vi "Find Execution Tests From AllTests.vi"(8 "error in":errorcluster, 10 "Test Tags to Execute":string[](array[string]), 11 "AllTests":refnum<class>[](array[class])) -> (0 "error out":errorcluster, 2 "ExecutionTests":refnum<class>[](array[class]))   [LabVIEW 2011, in "GraphicalTestRunner.lvlib"]
uses:
  GraphicalTestRunner.lvlib
  Classes/TestSuite/TestSuite.lvclass
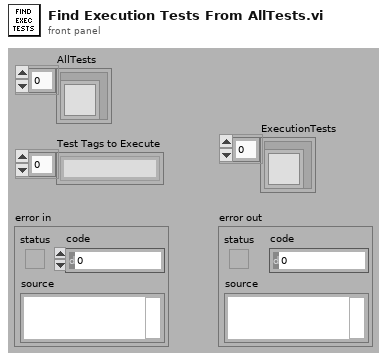
[diagram p1: front panel]
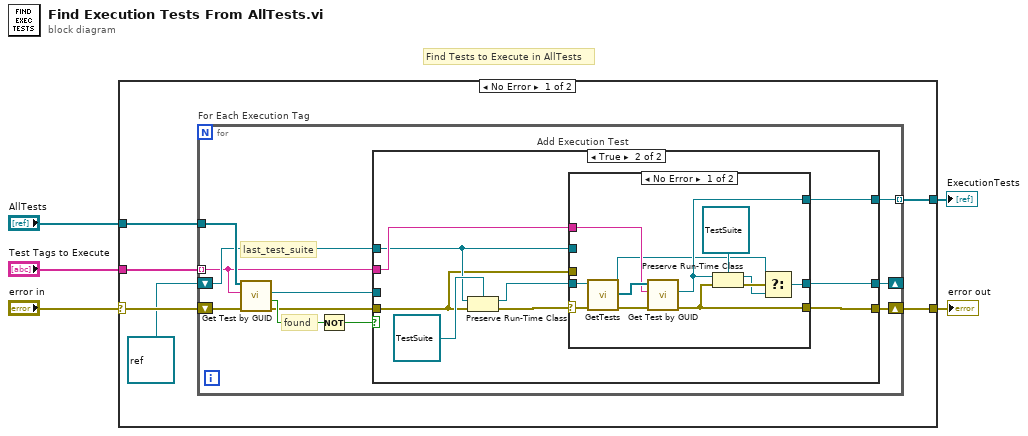
[diagram p0: block diagram]
diagram:
  # "Find Tests to Execute in AllTests"
  n1 = case shown="No Error" "error in" {
    selector: "error in" -> [w8 w49]
    tunnel: "AllTests" -> [w11 w48]
    tunnel: [w10 w48] -> w2
    tunnel: "Test Tags to Execute" -> [w9 _]
    tunnel: [w7 w49] -> w5
    frame No Error {
      n2 = for "For Each Execution Tag" {
        tunnel: w11 -> [w22]
        tunnel: [w19] -> w10 mode=indexing
        tunnel: w9 -> [w20] mode=indexing
        shift-right: [w18] -> _
        shift-left: refnum<class> refnum ("Test") -> [w21]
        shift-right: [w16] -> w7
        shift-left: w8 -> [w17]
        # "found"
        # "last_test_suite"
        n3 = call "Get Test by GUID.vi"("error in"=w17, "GUID"=w20, "AllTests"=w22) -> ("error out"=w13:errorcluster, "Found"=w15:bool, "Test"=w14:refnum<class>)  [unwired: 6 in]
        n4 = Not(x=w15) -> (.not. x?=w12:bool)
        n5 = case "Add Execution Test" shown="True" w12 {
          tunnel: [w24 w30] -> w19
          tunnel: w14 -> [w24 _]
          tunnel: w21 -> [_ w28]
          tunnel: w20 -> [_ w31]
          tunnel: [w24 w27] -> w18
          tunnel: w13 -> [w23 w25]
          tunnel: [w23 w26] -> w16
          frame False {
            # "May need to throw error\n\nThis means that a TestTag that we want to execute\nis not in \"AllTests\" --> user probably needs to reload hierarchy"
          }
          frame True {
            n6 = Preserve Run-Time Class(object in=w28, error in=w25, 2:refnum<class "TestSuite.lvclass"> refnum ("TestSuite in")) -> (object out=w32:refnum<class "TestSuite.lvclass">, error out=w29:errorcluster)
            n7 = case shown="No Error" w29 {
              selector: w29 -> [w36 _]
              tunnel: w32 -> [w45 _]
              tunnel: w31 -> [w43 _]
              tunnel: [w41 w47] -> w30
              tunnel: w28 -> [_ w47]
              tunnel: [w37 w47] -> w27
              tunnel: [w34 w46] -> w26
              tunnel: w25 -> [_ w46]
              frame No Error {
                n8 = call-dynamic "GetTests.vi"("error in (no error)"=w36, "TestSuite in"=w45) -> ("error out"=w35:errorcluster, "tests"=w44:refnum<class>[], "TestSuite in"=w39:refnum<class "TestSuite.lvclass">)  [unwired: 7 in]
                n9 = call "Get Test by GUID.vi"("error in"=w35, "GUID"=w43, "AllTests"=w44) -> ("error out"=w34:errorcluster, "Test"=w41:refnum<class>)  [unwired: 6 in, 1 out]
                n10 = Preserve Run-Time Class(object in=w41, error in=w34, 2:refnum<class "TestSuite.lvclass"> refnum ("TestSuite in")) -> (object out=w38:refnum<class "TestSuite.lvclass">, error out=w40:errorcluster)
                n11 = Select(t=w39, s=w40, f=w38) -> (s? t:f=w37:refnum<class "TestSuite.lvclass">)
              }
              frame Error {
              }
            }
          }
        }
      }
    }
    frame Error {
    }
  }
  "error out" <- w5
  "ExecutionTests" <- w2
